vi "get axis names.vi"(7 "Subsystem 1, 2, 3":i32=2, 10 "Axes":T1[](array[typedef]) items=["X"=1, "Y"=2, "Z"=3, "T"=4], 11 "Lookup Table":T2(array[cluster])) -> (3 "mmWave Names":string[](array[string]))   [LabVIEW 2019]
uses:
  <instrlib>/Velmex VXM/Public/VXM Axis.ctl
  <instrlib>/Velmex VXM/Velmex VXM.lvlib
panel:
  in  "Axis (1..4)":T1=1 items=["X"=1, "Y"=2, "Z"=3, "T"=4]
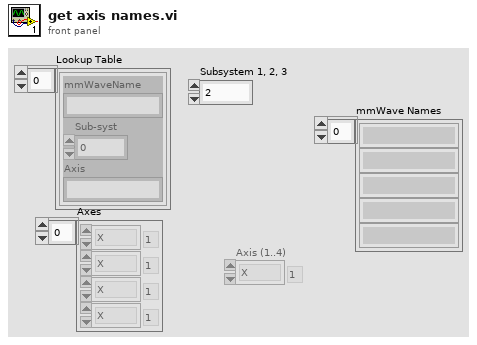
[diagram p1: front panel]
types:
  T1 = typedef "Velmex VXM.lvlib/VXM Axis.ctl" = u16
  T2 = cluster{"mmWaveName":string, "Sub-syst":i32, "Axis":string}[]
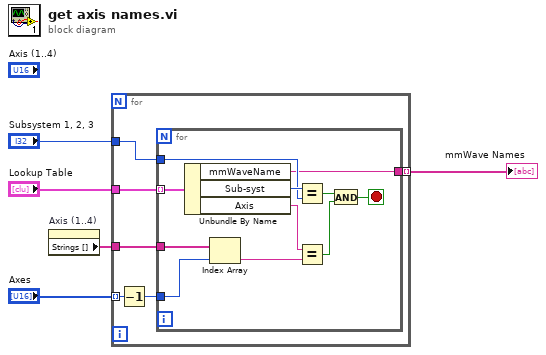
[diagram p0: block diagram]
diagram:
  n1 = property on="Axis (1..4)" class="Ring (strict)"() -> ("Strings []"=w3:string[])  [unwired: 2 in, 2 out]
  n2 = for {
    tunnel: "Axes" -> [w9] mode=indexing
    tunnel: "Lookup Table" -> [w11]
    tunnel: w3 -> [w10]
    tunnel: "Subsystem 1, 2, 3" -> [w8]
    tunnel: [w7] -> w1 mode=indexing
    n3 = Decrement(x=w9) -> (x-1=w6:T1)
    n4 = for {
      tunnel: w11 -> [w22] mode=indexing
      tunnel: w10 -> [w21]
      tunnel: w6 -> [w20]
      tunnel: w8 -> [w16]
      tunnel: [w12] -> w7
      stop <- w13 stop-if-true
      n5 = Unbundle By Name(w22) -> ("mmWaveName"=w12:string, "Sub-syst"=w17:i32, "Axis"=w19:string)
      n6 = Index Array(array=w21, index=w20) -> (element=w18:string)
      n7 = Equal?(x=w17, y=w16) -> (x = y?=w15:bool)
      n8 = Equal?(x=w19, y=w18) -> (x = y?=w14:bool)
      n9 = And(x=w15, y=w14) -> (x .and. y?=w13:bool)
    }
  }
  "mmWave Names" <- w1
